vi "CMD DoSomething.vi"(8 "error in (no error)":errorcluster, 11 "DbgTimers in":refnum<class "DbgTimers.lvclass">) -> (0 "error out":errorcluster, 3 "DbgTimers out":refnum<class "DbgTimers.lvclass">)   [LabVIEW 2017, in "DbgTimers.lvclass"]
doc: "Developed by Kevin Thompson\nkevin@thompsonengineering.net\n\nCopyright 2018-2020\nThompson Engineering, LLC"
uses:
  DbgTimers.lvclass
  DataTypes/AsynCmd_DbgTimers--enum.ctl
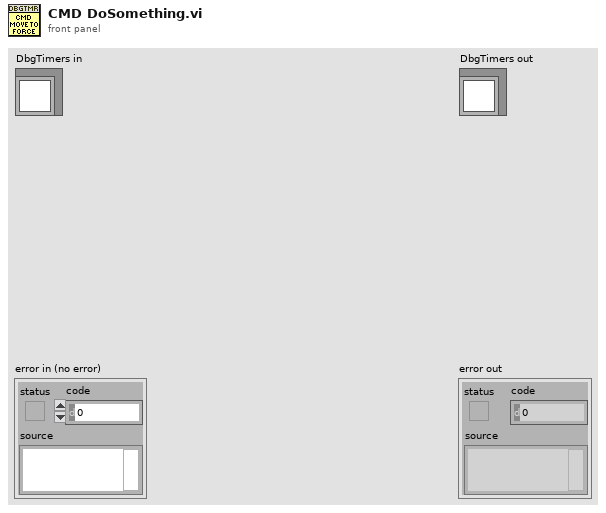
[diagram p1: front panel]
types:
  T1 = typedef "DbgTimers.lvclass/AsynCmd_DbgTimers--enum.ctl" = enum16{"DbgTimers.EnMsTickLogging", "DbgTimers.SetLogFolder"}
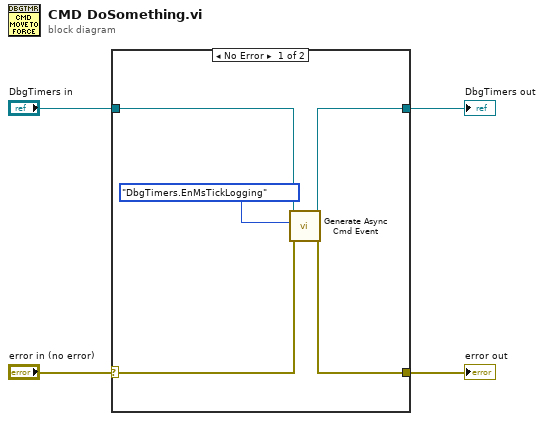
[diagram p0: block diagram]
diagram:
  n1 = case shown="No Error" "error in (no error)" {
    selector: "error in (no error)" -> [w7 w11]
    tunnel: [w6 w11] -> w3
    tunnel: [w8 w10] -> w1
    tunnel: "DbgTimers in" -> [w9 w10]
    frame No Error {
      n2 = call "Generate Async Cmd Event.vi"("error in (no error)"=w7, "AsyncCmd"=AsynCmd_DbgTimers--enum."DbgTimers.EnMsTickLogging", "DbgTimers in"=w9) -> ("error out"=w6:errorcluster, "DbgTimers out"=w8:refnum<class "DbgTimers.lvclass">)  [unwired: 7 in]
    }
    frame Error {
    }
  }
  "error out" <- w3
  "DbgTimers out" <- w1
